vi "Parse.vi"(8 "error in (no error)":errorcluster, 9 "channel blocks":T1[](array[typedef]) {"count" format="%d elements"; "First Channel Descriptor"."base address" format="%016x"; "First Channel Descriptor"."Channel Parameters"."offset" format="%d bytes"}, 10 "Buffer in":refnum<class "DSF.Engine.Memory.Buffer.lvclass">, 11 "Buffer Converter in":refnum<class "Buffer Converter.lvclass">) -> (0 "error out":errorcluster, 2 "Buffer out":refnum<class "DSF.Engine.Memory.Buffer.lvclass">, 3 "Buffer Converter out":refnum<class "Buffer Converter.lvclass">)   [LabVIEW 2017, in "Data Sharing Framework Engine.lvlib" / "Buffer Converter.lvclass"]
uses:
  Buffer Converter.lvclass
  old/dsf core/Source/Engine/Classes/Buffer/DSF.Engine.Memory.Buffer.lvclass
  old/dsf core/Source/Shared/Typedefs/DSF Runtime Channel Block Descriptor.ctl
  old/dsf core/Source/Shared/Typedefs/DSF Runtime Channel Descriptor.ctl
  old/dsf core/Source/Shared/Typedefs/DSF Runtime Channel Parameters.ctl
  Configuration/1.0.0/Public/Controls/DSF Data Type.ctl
  Buffer Converter.lvclass/Buffer Converter.ctl
  old/dsf core/Source/Engine/Classes/Buffer/DSF.Engine.Memory.Buffer.Read.1D.Bool.vi
  old/dsf core/Source/Engine/Classes/Buffer/DSF.Engine.Memory.Buffer.Read.1D.SGL.vi
  old/dsf core/Source/Engine/Classes/Buffer/DSF.Engine.Memory.Buffer.Read.1D.DBL.vi
  old/dsf core/Source/Engine/Classes/Buffer/DSF.Engine.Memory.Buffer.Read.1D.I8.vi
  old/dsf core/Source/Engine/Classes/Buffer/DSF.Engine.Memory.Buffer.Read.1D.I16.vi
  old/dsf core/Source/Engine/Classes/Buffer/DSF.Engine.Memory.Buffer.Read.1D.I32.vi
  old/dsf core/Source/Engine/Classes/Buffer/DSF.Engine.Memory.Buffer.Read.1D.I64.vi
  old/dsf core/Source/Engine/Classes/Buffer/DSF.Engine.Memory.Buffer.Read.1D.U8.vi
  old/dsf core/Source/Engine/Classes/Buffer/DSF.Engine.Memory.Buffer.Read.1D.U16.vi
  old/dsf core/Source/Engine/Classes/Buffer/DSF.Engine.Memory.Buffer.Read.1D.U32.vi
  old/dsf core/Source/Engine/Classes/Buffer/DSF.Engine.Memory.Buffer.Read.1D.U64.vi
  Data Sharing Framework Engine.lvlib
  Configuration/1.0.0/DSF Configuration API.lvlib
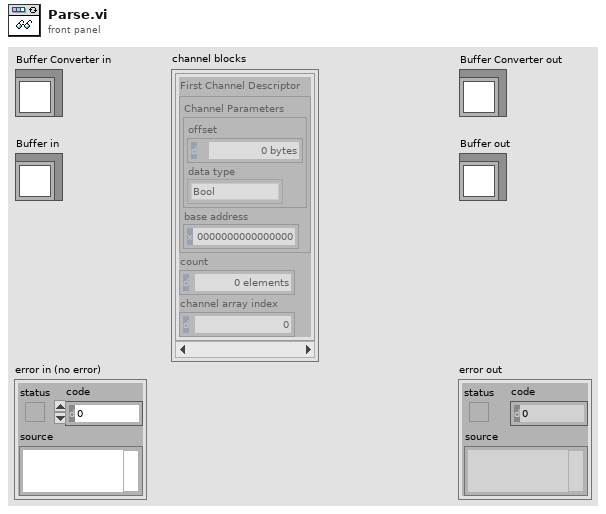
[diagram p1: front panel]
types:
  T1 = typedef "Data Sharing Framework Engine.lvlib/DSF Runtime Channel Block Descriptor.ctl" = cluster{"First Channel Descriptor":T2, "count":u64, "channel array index":u64}
  T2 = typedef "Data Sharing Framework Engine.lvlib/DSF Runtime Channel Descriptor.ctl" = cluster{"Channel Parameters":T3, "base address":u64}
  T3 = typedef "Data Sharing Framework Engine.lvlib/DSF Runtime Channel Parameters.ctl" = cluster{"offset":u64, "data type":T4}
  T4 = typedef "DSF Configuration API.lvlib/DSF Data Type.ctl" = enum8{"Bool", "SGL", "DBL", "I8", "I16", "I32", "I64", "U8", "U16", "U32", "U64"}
  T5 = typedef "Data Sharing Framework Engine.lvlib/DSF Runtime Type Buffers.ctl" = cluster{"Bool":bool[], "SGL":sgl[], "DBL":dbl[], "I8":i8[], "I16":i16[], "I32":i32[], "I64":i64[], "U8":u8[], "U16":u16[], "U32":u32[], "U64":u64[]}
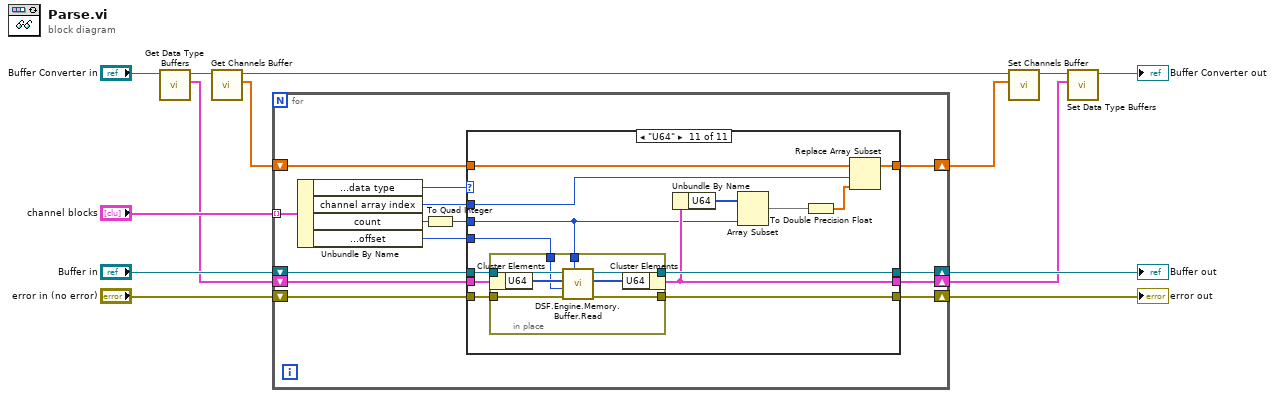
[diagram p0: block diagram]
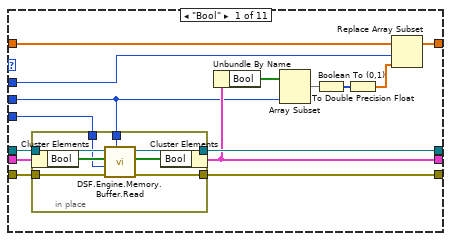
[diagram p2: hidden frame]
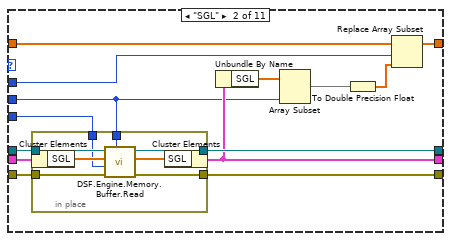
[diagram p3: hidden frame]
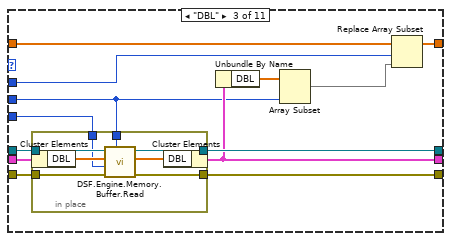
[diagram p4: hidden frame]
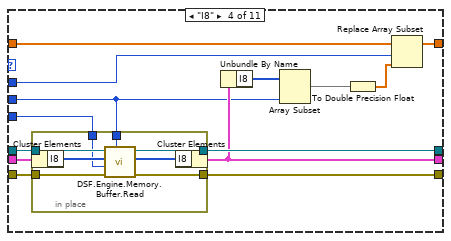
[diagram p5: hidden frame]
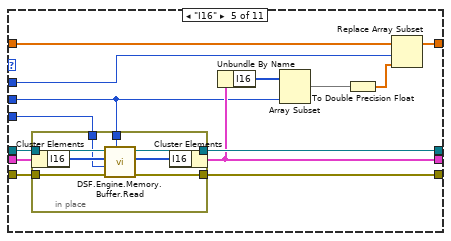
[diagram p6: hidden frame]
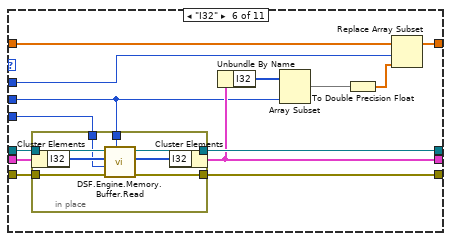
[diagram p7: hidden frame]
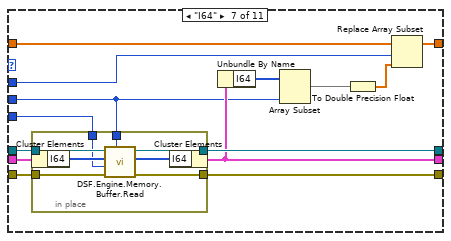
[diagram p8: hidden frame]
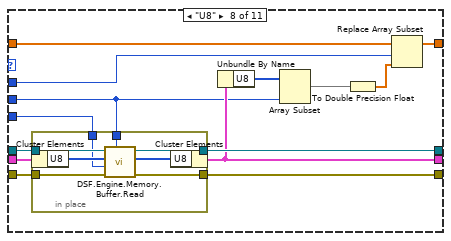
[diagram p9: hidden frame]
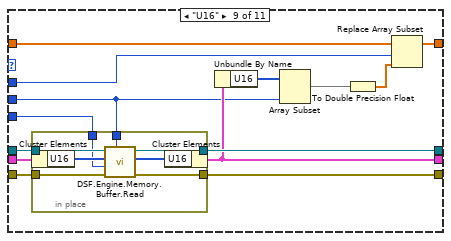
[diagram p10: hidden frame]
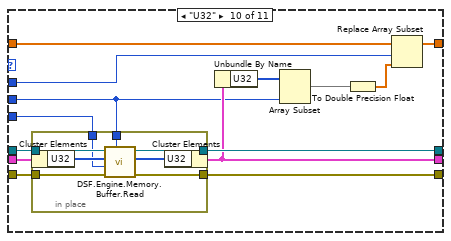
[diagram p11: hidden frame]
diagram:
  n1 = call "Get Data Type Buffers.vi"("Buffer Converter in"="Buffer Converter in") -> ("data type buffers"=w4:T5, "Buffer Converter out"=w5:refnum<class "Buffer Converter.lvclass">)  [unwired: 9 in]
  n2 = call "Get Channels Buffer.vi"("Buffer Converter in"=w5) -> ("channels buffer"=w8:dbl[], "Buffer Converter out"=w11:refnum<class "Buffer Converter.lvclass">)  [unwired: 9 in]
  n3 = for {
    tunnel: "channel blocks" -> [w21] mode=indexing
    shift-right: [w26] -> w13
    shift-left: "Buffer in" -> [w27]
    shift-right: [w20] -> w10
    shift-left: "error in (no error)" -> [w19]
    shift-right: [w15] -> w2
    shift-left: w4 -> [w16]
    shift-right: [w17] -> w7
    shift-left: w8 -> [w18]
    n4 = Unbundle By Name(w21) -> ("First Channel Descriptor.Channel Parameters.data type"=w28:T4, "channel array index"=w22:u64, "count"=w24:u64, "First Channel Descriptor.Channel Parameters.offset"=w25:u64)
    n5 = To Quad Integer(1:w24) -> (0:w23:i64)
    n6 = case shown="\"U64\"" w28 {
      tunnel: w27 -> [w43 w65 w86 w108 w130 w152 w174 w196 w218 w240 w262]
      tunnel: w19 -> [w42 w64 w85 w107 w129 w151 w173 w195 w217 w239 w261]
      tunnel: [w41 w63 w84 w106 w128 w150 w172 w194 w216 w238 w260] -> w20
      tunnel: [w40 w62 w83 w105 w127 w149 w171 w193 w215 w237 w259] -> w26
      tunnel: w16 -> [w39 w61 w82 w104 w126 w148 w170 w192 w214 w236 w258]
      tunnel: [w37 w59 w80 w102 w124 w146 w168 w190 w212 w234 w256] -> w15
      tunnel: w25 -> [w38 w60 w81 w103 w125 w147 w169 w191 w213 w235 w257]
      tunnel: w23 -> [w29 w53 w75 w96 w118 w140 w162 w184 w206 w228 w250]
      tunnel: w18 -> [w33 w57 w78 w100 w122 w144 w166 w188 w210 w232 w254]
      tunnel: [w32 w56 w77 w99 w121 w143 w165 w187 w209 w231 w253] -> w17
      tunnel: w22 -> [w30 w54 w76 w97 w119 w141 w163 w185 w207 w229 w251]
      frame "Bool" {
        n7 = in-place {
          in-place-border: w43 -> [w51]
          in-place-border: w42 -> [w50]
          in-place-border: [w49] -> w41
          in-place-border: w38 -> [w45]
          in-place-border: [w48] -> w40
          in-place-border: w29 -> [w44]
          n8 = in-place-cluster #1(w39) -> ("Bool"=w47:bool[])
          n9 = call-poly "DSF.Engine.Memory.Buffer.Read.vi"("count"=w44, "error in (no error)"=w50, "offset (0)"=w45, "buffer in"=w47, "Buffer in"=w51) -> ("error out"=w49:errorcluster, "buffer out"=w46:bool[], "Buffer out"=w48:refnum<class "DSF.Engine.Memory.Buffer.lvclass">)  [unwired: 3 in, 1 out]
          n10 = in-place-cluster #1("Bool"=w46) -> (w37:T5)
        }
        n11 = Unbundle By Name(w37) -> ("Bool"=w36:bool[])
        n12 = Array Subset(array=w36, length=w29) -> (w35:bool[])  [unwired: 1 in]
        n13 = Boolean To (0,1)(Boolean=w35) -> (0, 1=w34:i16[])
        n14 = To Double Precision Float(number=w34) -> (double precision float=w31:dbl[])
        n15 = Replace Array Subset(array=w33, new element=w31, index=w30) -> (w32:dbl[])
      }
      frame "SGL" {
        n16 = in-place {
          in-place-border: w65 -> [w73]
          in-place-border: w64 -> [w72]
          in-place-border: [w71] -> w63
          in-place-border: w60 -> [w67]
          in-place-border: [w70] -> w62
          in-place-border: w53 -> [w66]
          n17 = in-place-cluster #2(w61) -> ("SGL"=w69:sgl[])
          n18 = call-poly "DSF.Engine.Memory.Buffer.Read.vi"("count"=w66, "error in (no error)"=w72, "offset (0)"=w67, "buffer in"=w69, "Buffer in"=w73) -> ("error out"=w71:errorcluster, "buffer out"=w68:sgl[], "Buffer out"=w70:refnum<class "DSF.Engine.Memory.Buffer.lvclass">)  [unwired: 3 in, 1 out]
          n19 = in-place-cluster #2("SGL"=w68) -> (w59:T5)
        }
        n20 = Unbundle By Name(w59) -> ("SGL"=w58:sgl[])
        n21 = Array Subset(array=w58, length=w53) -> (w52:sgl[])  [unwired: 1 in]
        n22 = To Double Precision Float(number=w52) -> (double precision float=w55:dbl[])
        n23 = Replace Array Subset(array=w57, new element=w55, index=w54) -> (w56:dbl[])
      }
      frame "DBL" {
        n24 = in-place {
          in-place-border: w86 -> [w94]
          in-place-border: w85 -> [w93]
          in-place-border: [w92] -> w84
          in-place-border: w81 -> [w88]
          in-place-border: [w91] -> w83
          in-place-border: w75 -> [w87]
          n25 = in-place-cluster #3(w82) -> ("DBL"=w90:dbl[])
          n26 = call-poly "DSF.Engine.Memory.Buffer.Read.vi"("count"=w87, "error in (no error)"=w93, "offset (0)"=w88, "buffer in"=w90, "Buffer in"=w94) -> ("error out"=w92:errorcluster, "buffer out"=w89:dbl[], "Buffer out"=w91:refnum<class "DSF.Engine.Memory.Buffer.lvclass">)  [unwired: 3 in, 1 out]
          n27 = in-place-cluster #3("DBL"=w89) -> (w80:T5)
        }
        n28 = Unbundle By Name(w80) -> ("DBL"=w79:dbl[])
        n29 = Array Subset(array=w79, length=w75) -> (w74:dbl[])  [unwired: 1 in]
        n30 = Replace Array Subset(array=w78, new element=w74, index=w76) -> (w77:dbl[])
      }
      frame "I8" {
        n31 = in-place {
          in-place-border: w108 -> [w116]
          in-place-border: w107 -> [w115]
          in-place-border: [w114] -> w106
          in-place-border: w103 -> [w110]
          in-place-border: [w113] -> w105
          in-place-border: w96 -> [w109]
          n32 = in-place-cluster #4(w104) -> ("I8"=w112:i8[])
          n33 = call-poly "DSF.Engine.Memory.Buffer.Read.vi"("count"=w109, "error in (no error)"=w115, "offset (0)"=w110, "buffer in"=w112, "Buffer in"=w116) -> ("error out"=w114:errorcluster, "buffer out"=w111:i8[], "Buffer out"=w113:refnum<class "DSF.Engine.Memory.Buffer.lvclass">)  [unwired: 3 in, 1 out]
          n34 = in-place-cluster #4("I8"=w111) -> (w102:T5)
        }
        n35 = Unbundle By Name(w102) -> ("I8"=w101:i8[])
        n36 = Array Subset(array=w101, length=w96) -> (w95:i8[])  [unwired: 1 in]
        n37 = To Double Precision Float(number=w95) -> (double precision float=w98:dbl[])
        n38 = Replace Array Subset(array=w100, new element=w98, index=w97) -> (w99:dbl[])
      }
      frame "I16" {
        n39 = in-place {
          in-place-border: w130 -> [w138]
          in-place-border: w129 -> [w137]
          in-place-border: [w136] -> w128
          in-place-border: w125 -> [w132]
          in-place-border: [w135] -> w127
          in-place-border: w118 -> [w131]
          n40 = in-place-cluster #5(w126) -> ("I16"=w134:i16[])
          n41 = call-poly "DSF.Engine.Memory.Buffer.Read.vi"("count"=w131, "error in (no error)"=w137, "offset (0)"=w132, "buffer in"=w134, "Buffer in"=w138) -> ("error out"=w136:errorcluster, "buffer out"=w133:i16[], "Buffer out"=w135:refnum<class "DSF.Engine.Memory.Buffer.lvclass">)  [unwired: 3 in, 1 out]
          n42 = in-place-cluster #5("I16"=w133) -> (w124:T5)
        }
        n43 = Unbundle By Name(w124) -> ("I16"=w123:i16[])
        n44 = Array Subset(array=w123, length=w118) -> (w117:i16[])  [unwired: 1 in]
        n45 = To Double Precision Float(number=w117) -> (double precision float=w120:dbl[])
        n46 = Replace Array Subset(array=w122, new element=w120, index=w119) -> (w121:dbl[])
      }
      frame "I32" {
        n47 = in-place {
          in-place-border: w152 -> [w160]
          in-place-border: w151 -> [w159]
          in-place-border: [w158] -> w150
          in-place-border: w147 -> [w154]
          in-place-border: [w157] -> w149
          in-place-border: w140 -> [w153]
          n48 = in-place-cluster #6(w148) -> ("I32"=w156:i32[])
          n49 = call-poly "DSF.Engine.Memory.Buffer.Read.vi"("count"=w153, "error in (no error)"=w159, "offset (0)"=w154, "buffer in"=w156, "Buffer in"=w160) -> ("error out"=w158:errorcluster, "buffer out"=w155:i32[], "Buffer out"=w157:refnum<class "DSF.Engine.Memory.Buffer.lvclass">)  [unwired: 3 in, 1 out]
          n50 = in-place-cluster #6("I32"=w155) -> (w146:T5)
        }
        n51 = Unbundle By Name(w146) -> ("I32"=w145:i32[])
        n52 = Array Subset(array=w145, length=w140) -> (w139:i32[])  [unwired: 1 in]
        n53 = To Double Precision Float(number=w139) -> (double precision float=w142:dbl[])
        n54 = Replace Array Subset(array=w144, new element=w142, index=w141) -> (w143:dbl[])
      }
      frame "I64" {
        n55 = in-place {
          in-place-border: w174 -> [w182]
          in-place-border: w173 -> [w181]
          in-place-border: [w180] -> w172
          in-place-border: w169 -> [w176]
          in-place-border: [w179] -> w171
          in-place-border: w162 -> [w175]
          n56 = in-place-cluster #7(w170) -> ("I64"=w178:i64[])
          n57 = call-poly "DSF.Engine.Memory.Buffer.Read.vi"("count"=w175, "error in (no error)"=w181, "offset (0)"=w176, "buffer in"=w178, "Buffer in"=w182) -> ("error out"=w180:errorcluster, "buffer out"=w177:i64[], "Buffer out"=w179:refnum<class "DSF.Engine.Memory.Buffer.lvclass">)  [unwired: 3 in, 1 out]
          n58 = in-place-cluster #7("I64"=w177) -> (w168:T5)
        }
        n59 = Unbundle By Name(w168) -> ("I64"=w167:i64[])
        n60 = Array Subset(array=w167, length=w162) -> (w161:i64[])  [unwired: 1 in]
        n61 = To Double Precision Float(number=w161) -> (double precision float=w164:dbl[])
        n62 = Replace Array Subset(array=w166, new element=w164, index=w163) -> (w165:dbl[])
      }
      frame "U8" {
        n63 = in-place {
          in-place-border: w196 -> [w204]
          in-place-border: w195 -> [w203]
          in-place-border: [w202] -> w194
          in-place-border: w191 -> [w198]
          in-place-border: [w201] -> w193
          in-place-border: w184 -> [w197]
          n64 = in-place-cluster #8(w192) -> ("U8"=w200:u8[])
          n65 = call-poly "DSF.Engine.Memory.Buffer.Read.vi"("count"=w197, "error in (no error)"=w203, "offset (0)"=w198, "buffer in"=w200, "Buffer in"=w204) -> ("error out"=w202:errorcluster, "buffer out"=w199:u8[], "Buffer out"=w201:refnum<class "DSF.Engine.Memory.Buffer.lvclass">)  [unwired: 3 in, 1 out]
          n66 = in-place-cluster #8("U8"=w199) -> (w190:T5)
        }
        n67 = Unbundle By Name(w190) -> ("U8"=w189:u8[])
        n68 = Array Subset(array=w189, length=w184) -> (w183:u8[])  [unwired: 1 in]
        n69 = To Double Precision Float(number=w183) -> (double precision float=w186:dbl[])
        n70 = Replace Array Subset(array=w188, new element=w186, index=w185) -> (w187:dbl[])
      }
      frame "U16" {
        n71 = in-place {
          in-place-border: w218 -> [w226]
          in-place-border: w217 -> [w225]
          in-place-border: [w224] -> w216
          in-place-border: w213 -> [w220]
          in-place-border: [w223] -> w215
          in-place-border: w206 -> [w219]
          n72 = in-place-cluster #9(w214) -> ("U16"=w222:u16[])
          n73 = call-poly "DSF.Engine.Memory.Buffer.Read.vi"("count"=w219, "error in (no error)"=w225, "offset (0)"=w220, "buffer in"=w222, "Buffer in"=w226) -> ("error out"=w224:errorcluster, "buffer out"=w221:u16[], "Buffer out"=w223:refnum<class "DSF.Engine.Memory.Buffer.lvclass">)  [unwired: 3 in, 1 out]
          n74 = in-place-cluster #9("U16"=w221) -> (w212:T5)
        }
        n75 = Unbundle By Name(w212) -> ("U16"=w211:u16[])
        n76 = Array Subset(array=w211, length=w206) -> (w205:u16[])  [unwired: 1 in]
        n77 = To Double Precision Float(number=w205) -> (double precision float=w208:dbl[])
        n78 = Replace Array Subset(array=w210, new element=w208, index=w207) -> (w209:dbl[])
      }
      frame "U32" {
        n79 = in-place {
          in-place-border: w240 -> [w248]
          in-place-border: w239 -> [w247]
          in-place-border: [w246] -> w238
          in-place-border: w235 -> [w242]
          in-place-border: [w245] -> w237
          in-place-border: w228 -> [w241]
          n80 = in-place-cluster #10(w236) -> ("U32"=w244:u32[])
          n81 = call-poly "DSF.Engine.Memory.Buffer.Read.vi"("count"=w241, "error in (no error)"=w247, "offset (0)"=w242, "buffer in"=w244, "Buffer in"=w248) -> ("error out"=w246:errorcluster, "buffer out"=w243:u32[], "Buffer out"=w245:refnum<class "DSF.Engine.Memory.Buffer.lvclass">)  [unwired: 3 in, 1 out]
          n82 = in-place-cluster #10("U32"=w243) -> (w234:T5)
        }
        n83 = Unbundle By Name(w234) -> ("U32"=w233:u32[])
        n84 = Array Subset(array=w233, length=w228) -> (w227:u32[])  [unwired: 1 in]
        n85 = To Double Precision Float(number=w227) -> (double precision float=w230:dbl[])
        n86 = Replace Array Subset(array=w232, new element=w230, index=w229) -> (w231:dbl[])
      }
      frame "U64" {
        n87 = in-place {
          in-place-border: w262 -> [w270]
          in-place-border: w261 -> [w269]
          in-place-border: [w268] -> w260
          in-place-border: w257 -> [w264]
          in-place-border: [w267] -> w259
          in-place-border: w250 -> [w263]
          n88 = in-place-cluster #11(w258) -> ("U64"=w266:u64[])
          n89 = call-poly "DSF.Engine.Memory.Buffer.Read.vi"("count"=w263, "error in (no error)"=w269, "offset (0)"=w264, "buffer in"=w266, "Buffer in"=w270) -> ("error out"=w268:errorcluster, "buffer out"=w265:u64[], "Buffer out"=w267:refnum<class "DSF.Engine.Memory.Buffer.lvclass">)  [unwired: 3 in, 1 out]
          n90 = in-place-cluster #11("U64"=w265) -> (w256:T5)
        }
        n91 = Unbundle By Name(w256) -> ("U64"=w255:u64[])
        n92 = Array Subset(array=w255, length=w250) -> (w249:u64[])  [unwired: 1 in]
        n93 = To Double Precision Float(number=w249) -> (double precision float=w252:dbl[])
        n94 = Replace Array Subset(array=w254, new element=w252, index=w251) -> (w253:dbl[])
      }
    }
  }
  "error out" <- w10
  "Buffer out" <- w13
  n95 = call "Set Channels Buffer.vi"("channels buffer"=w7, "Buffer Converter in"=w11) -> ("Buffer Converter out"=w3:refnum<class "Buffer Converter.lvclass">)  [unwired: 9 in]
  n96 = call "Set Data Type Buffers.vi"("data type buffers"=w2, "Buffer Converter in"=w3) -> ("Buffer Converter out"=→"Buffer Converter out":refnum<class "Buffer Converter.lvclass">)  [unwired: 9 in]
